vi "Error Query.vi"(8 "error":errorcluster, 11 "VISA":refnum<visa-resource-name>) -> (0 "error out":errorcluster, 1 "Error Message":string, 2 "Error Number":i32, 3 "VISA out":refnum<visa-resource-name>)   [LabVIEW 2023, in "TDK-Lambda GEN LAN Series.lvlib"]
doc: "Reads an error code and a message from the instrument's error queue (query SYST:ERR?\"). Any instrument error is passed to the \"error out\" cluster as a VISA custom error. \n\nNote: This VI is called automatically by most driver VIs so it is usually *not* necessary to call this in an application.\n\nSee \"TDK-Lambda GEN LAN Readme.rtf\" in the driver project to understand the conversion from a system error code (+307 to -222) to VISA error code (-1074001663 to -1074001442)."
uses:
  TDK-Lambda GEN LAN Series.lvlib
panel:
  # "TDK-Lambda Genesys \n LAN\n  DC Power Supplies"
  # "Read\n  SYSTEM:ERROR?"
  # "(c) 2019 TDK-Lambda.  ALL RIGHTS RESERVED."
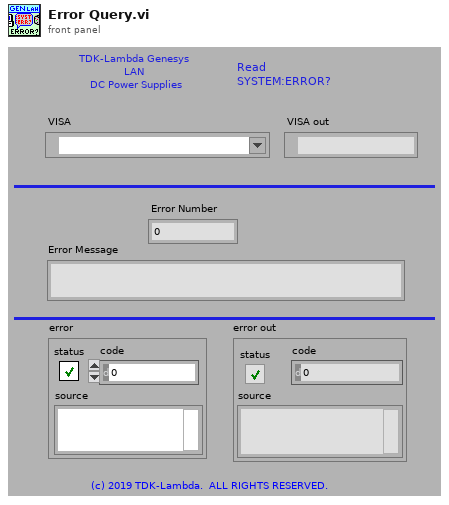
[diagram p1: front panel]
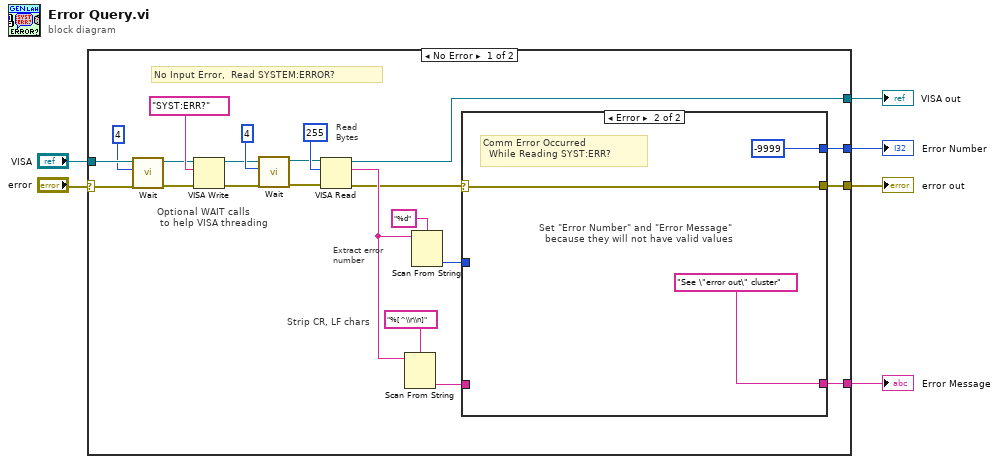
[diagram p0: block diagram]
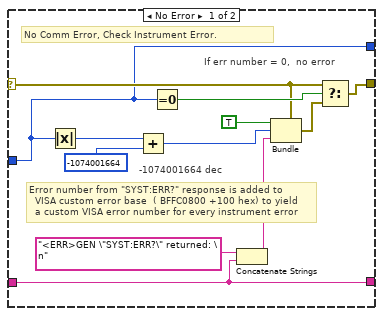
[diagram p2: hidden frame]
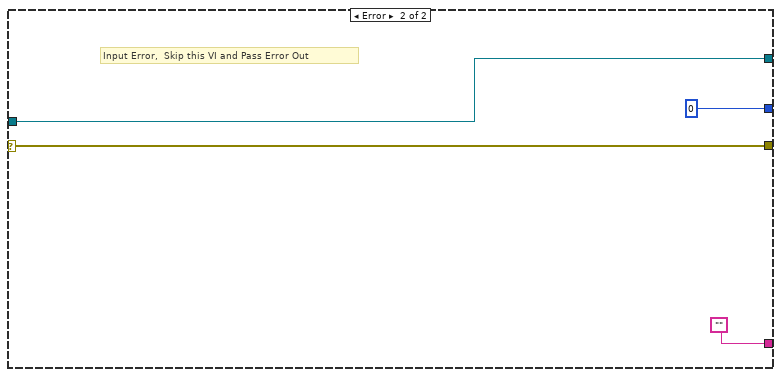
[diagram p3: hidden frame]
diagram:
  n1 = case shown="No Error" "error" {
    selector: "error" -> [w9 w44]
    tunnel: [w28 ""] -> w6
    tunnel: [w27 0] -> w5
    tunnel: [w18 w47] -> w4
    tunnel: "VISA" -> [w10 w47]
    tunnel: [w19 w44] -> w2
    frame No Error {
      # "Optional WAIT calls \n to help VISA threading"
      # "No Input Error,  Read SYSTEM:ERROR?"
      # "Extract error\nnumber"
      # "Read\nBytes"
      # "Strip CR, LF chars"
      n2 = call "Wait.vi"("error"=w9, "Delay (20 mS)"=u32 4, "VISA"=w10) -> ("error out"=w12:errorcluster, "VISA out"=w11:refnum<visa-resource-name>)  [unwired: 7 in]
      n3 = VISA Write(VISA resource name=w11, write buffer="SYST:ERR?", error in (no error)=w12) -> (VISA resource name out=w16:refnum<visa-resource-name>, error out=w14:errorcluster)  [unwired: 1 out]
      n4 = call "Wait.vi"("error"=w14, "Delay (20 mS)"=u32 4, "VISA"=w16) -> ("error out"=w13:errorcluster, "VISA out"=w15:refnum<visa-resource-name>)  [unwired: 7 in]
      n5 = VISA Read(VISA resource name=w15, byte count=u32 255 ("byte count (0)"), error in (no error)=w13) -> (VISA resource name out=w18:refnum<visa-resource-name>, read buffer=w21:string, error out=w7:errorcluster)  [unwired: 1 out]
      n6 = Scan From String(format string="%[^\\r\\n]", input string=w21) -> (output 1=w20:string)  [unwired: 3 in, 3 out]
      n7 = Scan From String(format string="%d", input string=w21) -> (output 1=w24:i32)  [unwired: 3 in, 3 out]
      n8 = case shown="Error" w7 {
        selector: w7 -> [w33 w41]
        tunnel: [w37 w41] -> w19
        tunnel: [w34 "See \"error out\" cluster" ("format string")] -> w28
        tunnel: [w32 -9999] -> w27
        tunnel: w24 -> [w32 _]
        tunnel: w20 -> [w34 _]
        frame No Error {
          # "No Comm Error, Check Instrument Error."
          # "Error number from \"SYST:ERR?\" response is added to \n  VISA custom error base  ( BFFC0800 +100 hex) to yield  \n  a custom VISA error number for every instrument error"
          # "-1074001664 dec"
          # "If err number = 0,  no error"
          n9 = Absolute Value(x=w32) -> (abs(x)=w31:i32)
          n10 = Add(x=w31, y=-1074001664) -> (x+y=w29:i32)
          n11 = Equal To 0?(x=w32) -> (x = 0?=w35:bool)
          n12 = Concatenate Strings("<ERR>GEN \"SYST:ERR?\" returned: \n" ("Source"), w34) -> (w39:string)
          n13 = Bundle(cluster=w33, "status"=TRUE ("Status"), "code"=w29, "source"=w39) -> (w38:errorcluster)
          n14 = Select(t=w33, s=w35, f=w38) -> (s? t:f=w37:errorcluster)
        }
        frame Error {
          # "Set \"Error Number\" and \"Error Message\"\n  because they will not have valid values"
          # "Comm Error Occurred  \n  While Reading SYST:ERR?"
        }
      }
    }
    frame Error {
      # "Input Error,  Skip this VI and Pass Error Out"
    }
  }
  "Error Message" <- w6
  "Error Number" <- w5
  "VISA out" <- w4
  "error out" <- w2
